vi "ReadWrite.vi"(8 "error in (no error)":errorcluster, 9 "Code":string, 11 "Python":T1) -> (0 "error out":errorcluster, 2 "Reply":string)   [LabVIEW 2021]
uses:
  Downloads/CEEO-smartmotors-main/SmartMotorUI/UI_Test_2.18.22/SerialVIs/PythonCtrl.ctl
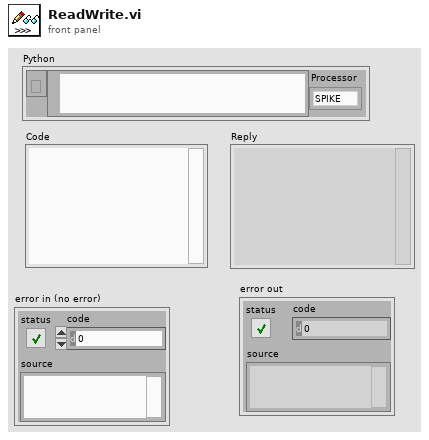
[diagram p1: front panel]
types:
  T1 = typedef "PythonCtrl.ctl" = cluster{"session":refnum<k35>, "PyPath":path, "Processor":enum16{"SPIKE", "Pi", "Pi_ssh"}}
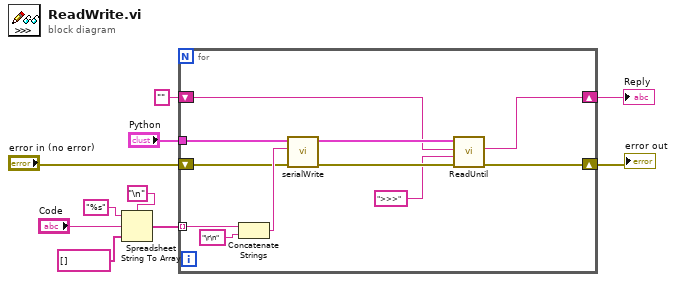
[diagram p0: block diagram]
diagram:
  n1 = Spreadsheet String To Array(delimiter (Tab)="\n", format string="%s", spreadsheet string="Code", array type (2D Dbl)=string[] []) -> (array=w10:string[])
  n2 = for {
    tunnel: "Python" -> [w15]
    tunnel: w10 -> [w18] mode=indexing
    shift-right: [w13] -> w3
    shift-left: "" -> [w14]
    shift-right: [w11] -> w1
    shift-left: "error in (no error)" -> [w12]
    n3 = Concatenate Strings(w18, "\r\n" ("delimiter (Tab)")) -> (w17:string)
    n4 = call "serialWrite.vi"("error in (no error)"=w12, "text"=w17, "Python"=w15) -> ("error out"=w20:errorcluster)  [unwired: 7 in, 1 out]
    n5 = call "ReadUntil.vi"("error in (no error)"=w20, "EOL"=">>>" ("regular expression"), "Console in"=w14, "Python"=w15) -> ("error out"=w11:errorcluster, "Console out"=w13:string)  [unwired: 6 in]
  }
  "Reply" <- w3
  "error out" <- w1
